vi "Read Valid Test Numbers.vi"(8 "error in (no error)":errorcluster, 11 "Test Group in":refnum<class "Test Group.lvclass">) -> (0 "error out":errorcluster, 2 "Valid Test Numbers":i32[](array[numeric]), 3 "Test Group out":refnum<class "Test Group.lvclass">)   [LabVIEW 2018, in "Test Number and Bin Generator.lvlib" / "Test Group.lvclass"]
uses:
  Test Group.lvclass
  Test Group.lvclass/Test Group.ctl
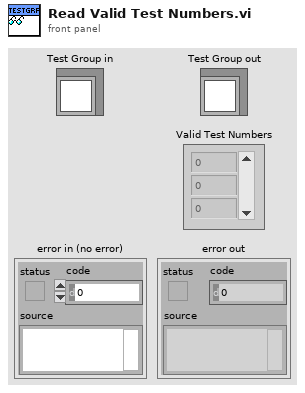
[diagram p1: front panel]
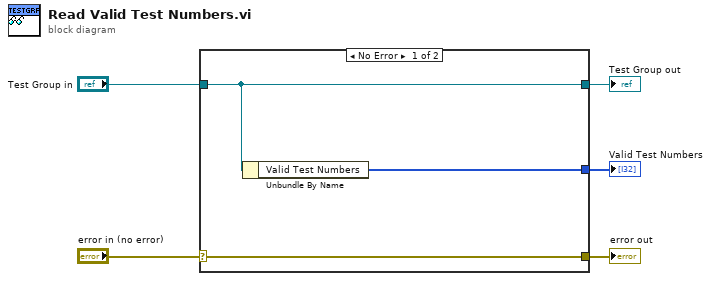
[diagram p0: block diagram]
diagram:
  n1 = case shown="No Error" "error in (no error)" {
    selector: "error in (no error)" -> [w8 w9]
    tunnel: [w8 w9] -> w4
    tunnel: [w7 w10] -> w2
    tunnel: "Test Group in" -> [w7 w10]
    tunnel: [w6 _] -> w1
    frame No Error {
      n2 = Unbundle By Name(w7) -> ("Valid Test Numbers"=w6:i32[])
    }
    frame Error {
    }
  }
  "error out" <- w4
  "Test Group out" <- w2
  "Valid Test Numbers" <- w1
